vi "Parse Kasli Request.vi"(8 "error in (no error)":errorcluster, 10 "Message part":string, 11 "TCP Server in":refnum<class "TCP Server.lvclass">) -> (0 "error out":errorcluster, 1 "uService Class Name":string, 2 "uService ID":string, 3 "TCP Server Msg Actions":T1)   [LabVIEW 2026, in "TALOS.lvlib" / "TCP Server.lvlib" / "TCP Server.lvclass"]
uses:
  TCP Server.lvclass
  TCP Server Msg Actions.ctl
  Ancestor/Ancestor/Ancestor.lvclass/Ancestor.ctl
  d942f059-2b1b-4d9b-ba76-91ff54e3f6fc.vi
  <vilib>/Utility/error.llb/Trim Whitespace (string).vi
  <vilib>/AdvancedString/Delimited String to 1D String Array (string).vi
  FGV/Error Memory/Get Error Description.vi
  Support VIs/Get PC name.vi
  Ancestor/Ancestor/Read ID.vi
  Support VIs/Get Class Name.vi
  <vilib>/Utility/error.llb/Clear Errors.vi
  <vilib>/Utility/error.llb/Trim Whitespace One-Sided.vi
  FGV/Error Memory/Error Memory Core.vi
  Support VIs/Circus Root Path.vi
  FGV/Error Memory/Error Crt Lvl checker.vi
  FGV/Error Memory/Error Memory Core.vi/40c8088d-b597-4017-91af-faa98e00292e.vi
  FGV/Error Memory/Error Memory Core.vi/d4a3ab98-063c-4e44-b43d-fbdcfe6c2be2.vi
  Support VIs/Global Memory.vi
  <vilib>/Utility/LVClass/Get LV Class Name.vi
  Support VIs/Is in Packed Library.vi
  Support VIs/TALOS Root path.vi
  Support VIs/Read CSV worksheet.vi
  Support VIs/Global Constants.vi
  <vilib>/Utility/error.llb/General Error Handler.vi
  <vilib>/Comparison/Equal/Equal Functor/Equal Functor.lvclass
  Ancestor/Ancestor/Ancestor.lvclass
  TALOS.lvlib
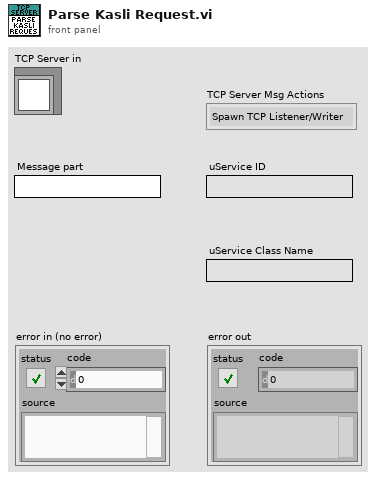
[diagram p1: front panel]
types:
  T1 = typedef "TALOS.lvlib/TCP Server.lvlib/TCP Server.lvclass/TCP Server Msg Actions.ctl" = enum16{"Spawn TCP Listener/Writer", "External Error", "I Exist", "Who the hell is this guy?", "Do nothing", "Are you the Bearer", "Farewell", "External Message"}
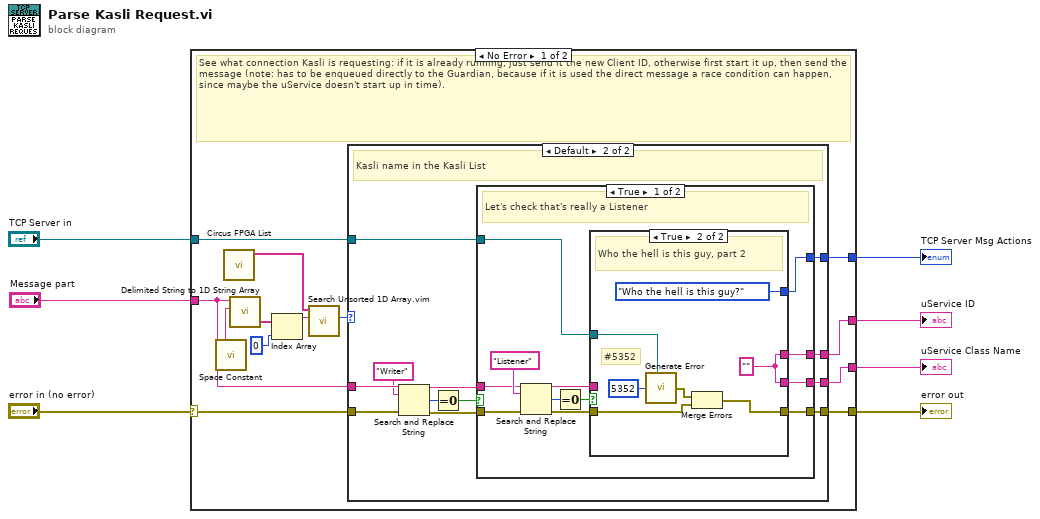
[diagram p0: block diagram]
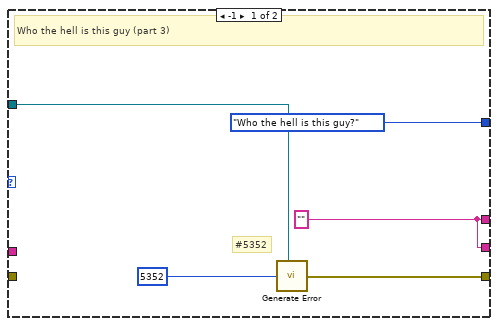
[diagram p2: hidden frame]
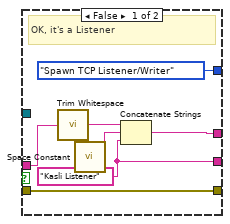
[diagram p3: hidden frame]
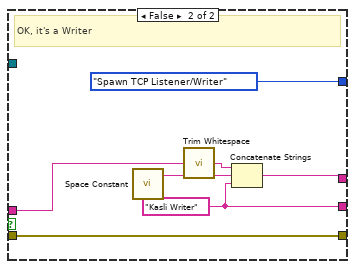
[diagram p4: hidden frame]
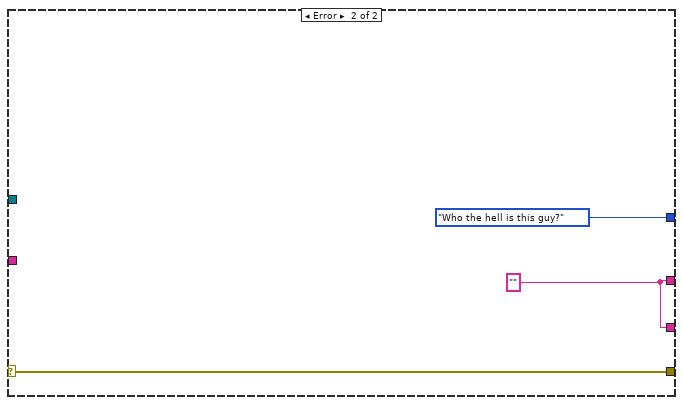
[diagram p5: hidden frame]
diagram:
  n1 = case shown="No Error" "error in (no error)" {
    selector: "error in (no error)" -> [w20 w72]
    tunnel: "Message part" -> [w19 _]
    tunnel: [w12 w73] -> w5
    tunnel: "TCP Server in" -> [w11 _]
    tunnel: [w10 w72] -> w3
    tunnel: [w9 w73] -> w2
    tunnel: [w8 TCP_Server_Msg_Actions."Who the hell is this guy?"] -> w1
    frame No Error {
      # "See what connection Kasli is requesting: if it is already running, just send it the new Client ID, otherwise first start it up, then send the message (note: has to be enqueued directly to the Guardian, because if it is used the direct message a race condition can happen, since maybe the uService doesn't start up in time)."
      n2 = call <vilib>:"Space Constant.vi"() -> ("String"=w18:string)
      n3 = call "Circus FPGA List.vi"() -> ("FPGA List out"=w13:string[])  [unwired: 10 in, 1 out]
      n4 = call-poly <vilib>:"Delimited String to 1D String Array.vi"("delimiter"=w18, "delimited string"=w19) -> ("string array"=w16:string[])  [unwired: 9 in]
      n5 = Index Array(array=w16, index=0) -> (element=w15:string)
      n6 = call "Search Unsorted 1D Array.vim"("element"=w15, "unsorted 1D array"=w13) -> ("index of element"=w14:i32)  [unwired: 9 in]
      n7 = case shown="Default" w14 {
        tunnel: [w22 w37] -> w9
        tunnel: [w23 w36] -> w10
        tunnel: w11 -> [w24 w35]
        tunnel: [w22 w34] -> w12
        tunnel: w19 -> [_ w32]
        tunnel: w20 -> [_ w30]
        tunnel: [TCP_Server_Msg_Actions."Who the hell is this guy?" w26] -> w8
        frame -1 {
          w22 = "" ("uService ID")
          # "#5352"
          # "Who the hell is this guy (part 3)"
          n8 = call "Generate Error.vi"("Class"=w24, "Error Code"=5352) -> ("error out"=w23:errorcluster)  [unwired: 5 in]
        }
        frame Default {
          # "Kasli name in the Kasli List"
          n9 = Search and Replace String(input string=w32, search string="Writer", error in=w30) -> (result string=w28:string, number of replacements=w33:i32, error out=w27:errorcluster)  [unwired: 5 in, 1 out]
          n10 = Equal To 0?(x=w33) -> (x = 0?=w29:bool)
          n11 = case shown="True" w29 {
            tunnel: [w49 w69] -> w34
            tunnel: [w44 w68] -> w37
            tunnel: w27 -> [w46 w70]
            tunnel: [w41 w70] -> w36
            tunnel: w28 -> [w45 w65]
            tunnel: w35 -> [w42 _]
            tunnel: [w38 TCP_Server_Msg_Actions."Spawn TCP Listener/Writer"] -> w26
            frame True {
              # "Let's check that's really a Listener"
              n12 = Search and Replace String(input string=w45, search string="Listener", error in=w46) -> (result string=w39:string, number of replacements=w48:i32, error out=w40:errorcluster)  [unwired: 5 in, 1 out]
              n13 = Equal To 0?(x=w48) -> (x = 0?=w43:bool)
              n14 = case shown="True" w43 {
                tunnel: [w55 w63] -> w49
                tunnel: [w54 w63] -> w44
                tunnel: w42 -> [_ w61]
                tunnel: [w56 w59] -> w41
                tunnel: w40 -> [w56 w58]
                tunnel: w39 -> [w51 _]
                tunnel: [TCP_Server_Msg_Actions."Spawn TCP Listener/Writer" TCP_Server_Msg_Actions."Who the hell is this guy?"] -> w38
                frame False {
                  w54 = "Kasli Listener" ("uService ID")
                  # "OK, it's a Listener"
                  n15 = call-poly <vilib>:"Trim Whitespace.vi"("string"=w51) -> ("trimmed string"=w52:string)  [unwired: 1 in]
                  n16 = call <vilib>:"Space Constant.vi"() -> ("String"=w53:string)
                  n17 = Concatenate Strings(w52, w53, w54) -> (w55:string)
                }
                frame True {
                  w63 = "" ("uService ID")
                  # "#5352"
                  # "Who the hell is this guy, part 2"
                  n18 = call "Generate Error.vi"("Class"=w61, "Error Code"=5352) -> ("error out"=w60:errorcluster)  [unwired: 5 in]
                  n19 = Merge Errors(w60, w58) -> (w59:errorcluster)
                }
              }
            }
            frame False {
              w68 = "Kasli Writer" ("uService ID")
              # "OK, it's a Writer"
              n20 = call <vilib>:"Space Constant.vi"() -> ("String"=w67:string)
              n21 = call-poly <vilib>:"Trim Whitespace.vi"("string"=w65) -> ("trimmed string"=w66:string)  [unwired: 1 in]
              n22 = Concatenate Strings(w66, w67, w68) -> (w69:string)
            }
          }
        }
      }
    }
    frame Error {
      w73 = "" ("uService ID")
    }
  }
  "uService ID" <- w5
  "error out" <- w3
  "uService Class Name" <- w2
  "TCP Server Msg Actions" <- w1
